vi "FGV-class check.vi"() -> ()   [LabVIEW 2018]
panel:
  in  "file path":path=path "C:/Users/BoasLab/Documents/Data/Alazar data/B-line/data/test.tif"
  out "Array 2":string[](array[string])
  out "Array":u32[](array[numeric])
  in  "Galvo HW Parameters":T1={"Analog Out Channel"="GalvoCtrl/ao0,GalvoCtrl/ao1", "Min Voltage"=-10.0, "Max Voltage"=10.0, "Pixel Clock Source"="/GalvoCtrl/PFI0", "Sample Rate"=1000.0, "Line Clock Out Ch"="GalvoCtrl/port0/line0"}
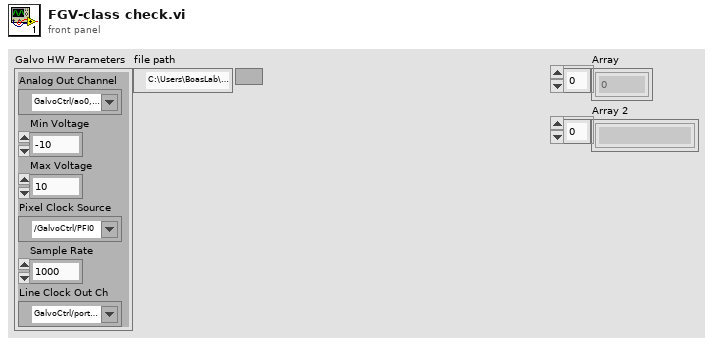
[diagram p1: front panel]
types:
  T1 = cluster{"Analog Out Channel":tag, "Min Voltage":dbl, "Max Voltage":dbl, "Pixel Clock Source":tag, "Sample Rate":dbl, "Line Clock Out Ch":tag}
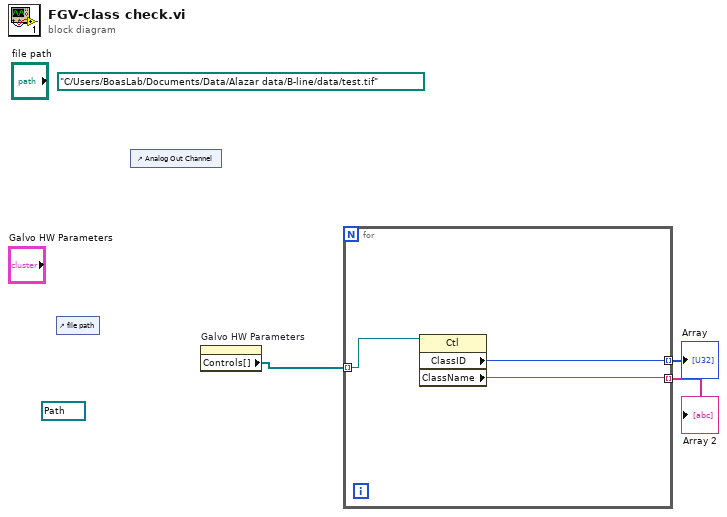
[diagram p0: block diagram]
diagram:
  (unwired) refnum<vi> refnum ("file path")
  (unwired) path "C:/Users/BoasLab/Documents/Data/Alazar data/B-line/data/test.tif" ("file path")
  n1 = control-ref of="file path"() -> ()  [unwired: 1 out]
  n2 = control-ref of="Analog Out Channel"() -> ()  [unwired: 1 out]
  n3 = property on="Galvo HW Parameters" class="Clust (strict)"() -> ("Controls[]"=w3:refnum<vi>[])  [unwired: 2 in, 2 out]
  n4 = for {
    tunnel: w3 -> [w6] mode=indexing
    tunnel: [w5] -> w2 mode=indexing
    tunnel: [w4] -> w1 mode=indexing
    n5 = property class="Ctl"(reference=w6) -> ("ClassID"=w5:u32, "ClassName"=w4:string)  [unwired: 1 in, 2 out]
  }
  "Array" <- w2
  "Array 2" <- w1
